vi "Lorentzian complex bg test Jacobian.vi"(3 "output control":T1, 4 "data":variant, 5 "X":dbl[](array[numeric]), 6 "a":dbl[](array[numeric])) -> (0 "error out":errorcluster, 1 "f'(X,a)":dbl[][](array[numeric]), 2 "f(X,a)":dbl[](array[numeric]))   [LabVIEW 2016]
doc: "Sum of three Gaussians, plus DC offset."
uses:
  <vilib>/gmath/NumericalOptimization/LM_output select.ctl
  <vilib>/gmath/NI_Gmath.lvlib
panel:
  out "Waveform Graph":dbl[][](graph)
  # "F0\nG\nA\nP\nX\nY"
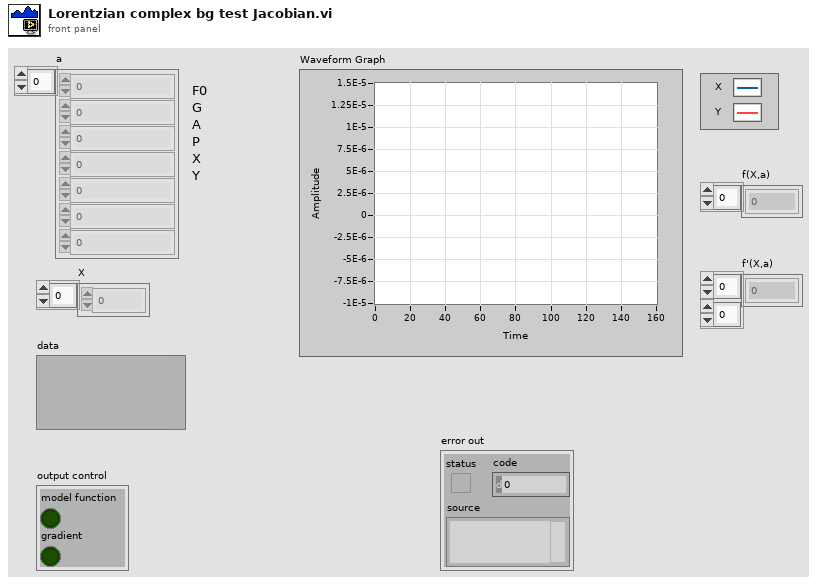
[diagram p1: front panel]
types:
  T1 = typedef "NI_Gmath.lvlib/LM_output select.ctl" = cluster{"model function":bool, "gradient":bool}
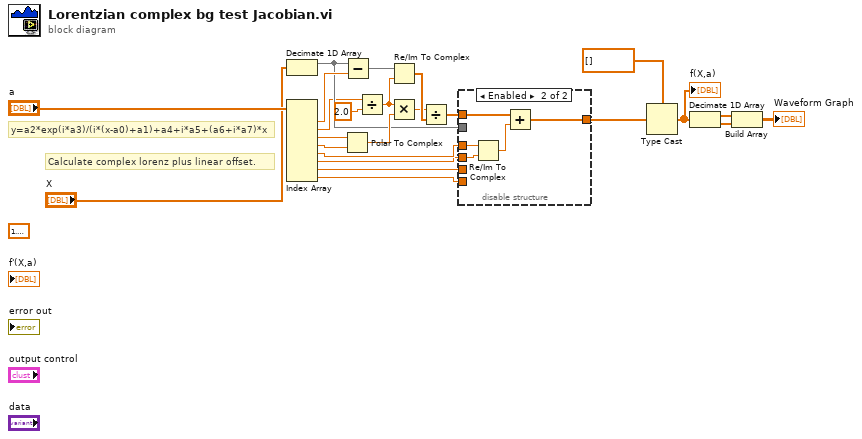
[diagram p0: block diagram]
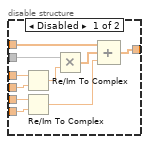
[diagram p2: hidden frame]
diagram:
  (unwired) 1.5707963267948966
  # "y=a2*exp(i*a3)/(i*(x-a0)+a1)+a4+i*a5+(a6+i*a7)*x"
  # "Calculate complex lorenz plus linear offset."
  n1 = Decimate 1D Array("X") -> (w11:dbl[])  [unwired: 1 out]
  n2 = Index Array(array="a") -> (element #1=w23:dbl, element #2=w6:dbl, element #3=w20:dbl, element #4=w19:dbl, element #5=w17:dbl, element #6=w16:dbl, element #7=w14:dbl, element #8=w13:dbl)  [unwired: 8 in]
  n3 = Polar To Complex(1:w19, 2:w20) -> (0:w22:cdb)
  n4 = Subtract(x=w11, y=w23) -> (x-y=w9:dbl[])
  n5 = Divide(x=w6, y=2.0) -> (x/y=w5:dbl)
  n6 = Re/Im To Complex(1:w5, 2:w9) -> (0:w21:cdb[])
  n7 = Multiply(x=w5, y=w22) -> (x*y=w8:cdb)
  n8 = Divide(x=w8, y=w21) -> (x/y=w12:cdb[])
  n9 = disable-structure shown="Enabled" {
    disable-tunnel: w17 -> [w34 w39]
    disable-tunnel: w16 -> [w33 w38]
    disable-tunnel: w14 -> [w30 _]
    disable-tunnel: w13 -> [w29 _]
    disable-tunnel: w12 -> [w27 w37]
    disable-tunnel: [w26 w36] -> w10
    disable-tunnel: w11 -> [w25 _]
    frame Disabled {
      n10 = Re/Im To Complex(1:w33, 2:w34) -> (0:w32:cdb)
      n11 = Re/Im To Complex(1:w29, 2:w30) -> (0:w28:cdb)
      n12 = Multiply(x=w25, y=w32) -> (x*y=w31:cdb[])
      n13 = Compound Arithmetic op=ADD(w27, w31, w28) -> (w26:cdb[])
    }
    frame Enabled {
      n14 = Re/Im To Complex(1:w38, 2:w39) -> (0:w35:cdb)
      n15 = Add(x=w37, y=w35) -> (x+y=w36:cdb[])
    }
  }
  n16 = Type Cast(type=dbl[] [], x=w10) -> (*(type *) &x=w4:dbl[])
  "f(X,a)" <- w4
  n17 = Decimate 1D Array(w4) -> (w3:dbl[], w2:dbl[])
  n18 = Build Array(w3, w2) -> (→"Waveform Graph":dbl[][])
